vi "Client.vi"() -> ()   [LabVIEW 2020]
panel:
  in  "stop":bool
  out "data out":string
  out "error out":errorcluster
  # "Cliente"
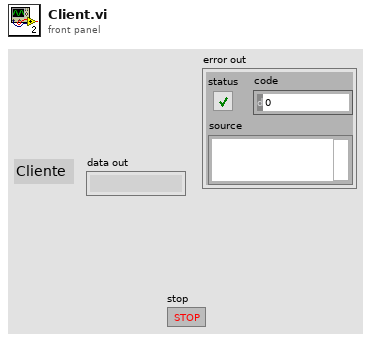
[diagram p1: front panel]
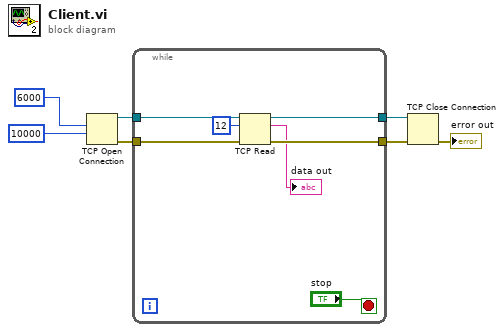
[diagram p0: block diagram]
diagram:
  n1 = TCP Open Connection(remote port or service name=u16 6000, timeout ms (60000)=10000) -> (connection ID=w7:refnum<k5>, error out=w5:errorcluster)  [unwired: 3 in]
  n2 = while {
    tunnel: w7 -> [w14]
    tunnel: [w13] -> w6
    tunnel: w5 -> [w12]
    tunnel: [w11] -> w4
    stop <- "stop" stop-if-true
    n3 = TCP Read(connection ID=w14, bytes to read=12, error in (no error)=w12) -> (connection ID out=w13:refnum<k5>, data out=→"data out":string, error out=w11:errorcluster)  [unwired: 2 in]
  }
  n4 = TCP Close Connection(connection ID=w6, error in (no error)=w4) -> (error out=→"error out":errorcluster)  [unwired: 1 in, 1 out]
